vi "save_max_p_Data.vi"(0 "Experiment Indicator":string, 1 "Cell details cluster":T3={"Cell Position"=16, "Cell Label"="", "Pixel to measure"=0, "Area (cm^2)"=0.126, "Variable"="", "Variable value"="", "Scan settings in queue"=0, "Light or dark"="", "Measurement Type"=""} {"Pixel to measure" items=["All", "1", "2", "3", "4", "5", "6", "7", "8"]}, 3 "Intensity (no. of suns)":string, 4 "Data Array":dbl[][](array[numeric]), 6 "Username":string, 7 "Scan settings":T1={"J-V scan"=TRUE, "J-t scan"=FALSE, "Min voltage (V)"=0.0, "Max voltage (V)"=1.4, "Step (V)"=0.01, "Measurement delay (ms)"=10.0, "1st scan FB-SC"=TRUE, "Inverted structure"=FALSE, "Stabilisation time (s)"=0.0, "Stabilisation mode"=0, "Stabilisation value (V or A) "=0.0, "Step time (s)"=1.0, "Integration time"=0, "Repeat light scans"=FALSE, "Stabilisation in the dark?"=FALSE, "J-t Min (V)"=0.0, "J-t Max (V)"=1.4, "J-t Step (V)"=0.01, "Max. power stabilisation"=FALSE, "J-t 1st scan FB-SC"=TRUE, "J-t Inverted structure"=FALSE, "Max power tracking"=FALSE, "Vmp (V)"=0.7, "Total stabilisation time (s)"=100.0, "J-t best pixel only"=0, "Max power best pixel only"=0, "Vmp from J-V scan"=FALSE, "No. of repeat scans"=2.0, "Only repeat for best pixel"=0, "Stabilisation time step (s)"=1.0, "Illumination conditions"=2, "Scan rate min (V/s)"=0.1, "Scan rate max (V/s)"=1.0, "No. of scan rate steps"=1.0, "Scan rate voltage step priority"=FALSE, "Scan rate measurement delay priority"=FALSE, "J-t Illumination conditions"=0, "Max P stab. Specific voltage"=FALSE} {"J-t Illumination conditions" items=["Light only", "Dark only", "Light then dark", "Dark then light"]; "No. of scan rate steps" min=1.0 step=1.0; "Illumination conditions" items=["Light only", "Dark only", "Light then dark", "Dark then light", "Light then dark then light", "Dark then light then dark"]; "Only repeat for best pixel" items=["only for best pixel", "for best 2 pixels", "for best 3 pixels", "for best 4 pixels", "for best 5 pixels", "for best 6 pixels", "for best 7 pixels", "for all pixels"]; "No. of repeat scans" min=1.0 step=1.0; "Max power best pixel only" items=["only the best pixel", "the best 2 pixels", "the best 3 pixels", "the best 4 pixels", "the best 5 pixels", "the best 6 pixels", "the best 7 pixels", "all pixels"]; "J-t best pixel only" items=["only the best pixel", "the best 2 pixels", "the best 3 pixels", "the best 4 pixels", "the best 5 pixels", "the best 6 pixels", "the best 7 pixels", "all pixels"]; "Integration time" items=["Fast", "Normal", "High Accuracy"]; "Stabilisation mode" items=["V", "I"]; "Measurement delay (ms)" min=10.0}, 10 "Date array":string[](array[string])) -> (14 "Master Log":string[][](table), 15 "File path for master log":path, 17 "File path for Jt data":path, 18 "File path for Jt image":path)   [LabVIEW 2016]
uses:
  TypeDefs/scan_settings.ctl
  TypeDefs/Settings Boolean.ctl
  <vilib>/Utility/file.llb/Write Delimited Spreadsheet (string).vi
  <vilib>/Utility/file.llb/Read Delimited Spreadsheet (string).vi
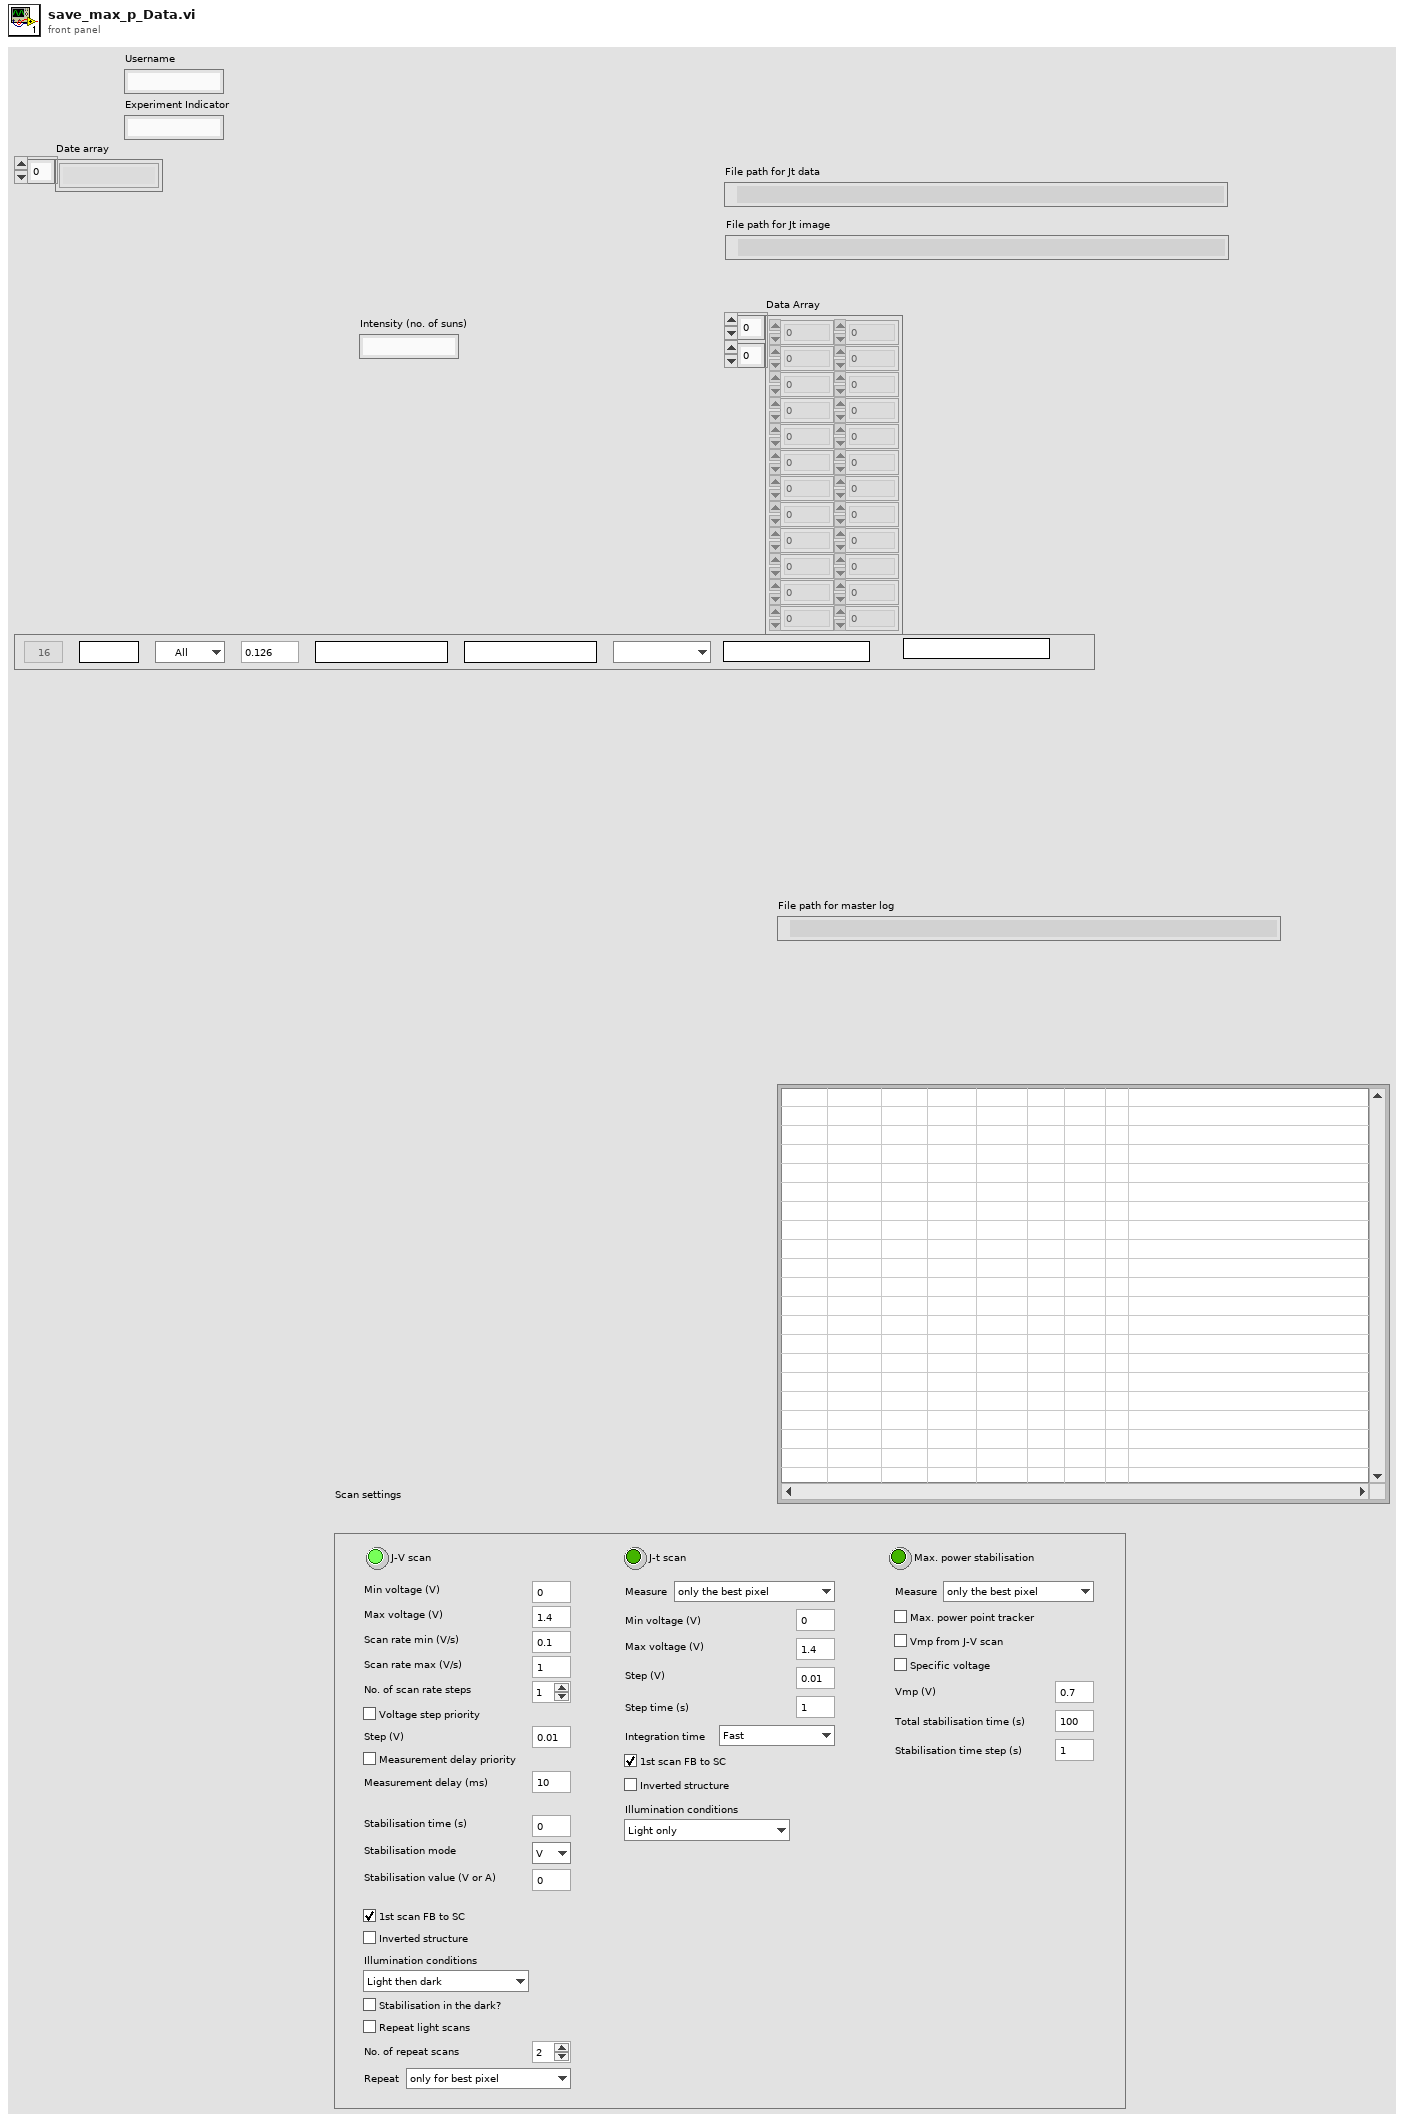
[diagram p1: front panel]
types:
  T1 = typedef "scan_settings.ctl" = cluster{"J-V scan":T2, "J-t scan":bool, "Min voltage (V)":dbl, "Max voltage (V)":dbl, "Step (V)":dbl, "Measurement delay (ms)":dbl, "1st scan FB-SC":bool, "Inverted structure":bool, "Stabilisation time (s)":dbl, "Stabilisation mode":u16, "Stabilisation value (V or A) ":dbl, "Step time (s)":dbl, "Integration time":u16, "Repeat light scans":bool, "Stabilisation in the dark?":bool, "J-t Min (V)":dbl, "J-t Max (V)":dbl, "J-t Step (V)":dbl, "Max. power stabilisation":bool, "J-t 1st scan FB-SC":bool, "J-t Inverted structure":bool, "Max power tracking":bool, "Vmp (V)":dbl, "Total stabilisation time (s)":dbl, "J-t best pixel only":u16, "Max power best pixel only":u16, "Vmp from J-V scan":bool, "No. of repeat scans":dbl, "Only repeat for best pixel":u16, "Stabilisation time step (s)":dbl, "Illumination conditions":u16, "Scan rate min (V/s)":dbl, "Scan rate max (V/s)":dbl, "No. of scan rate steps":dbl, "Scan rate voltage step priority":bool, "Scan rate measurement delay priority":bool, "J-t Illumination conditions":u16, "Max P stab. Specific voltage":bool}
  T2 = typedef "Settings Boolean.ctl" = bool
  T3 = cluster{"Cell Position":i32, "Cell Label":string, "Pixel to measure":u16, "Area (cm^2)":dbl, "Variable":string, "Variable value":string, "Scan settings in queue":u16, "Light or dark":string, "Measurement Type":string}
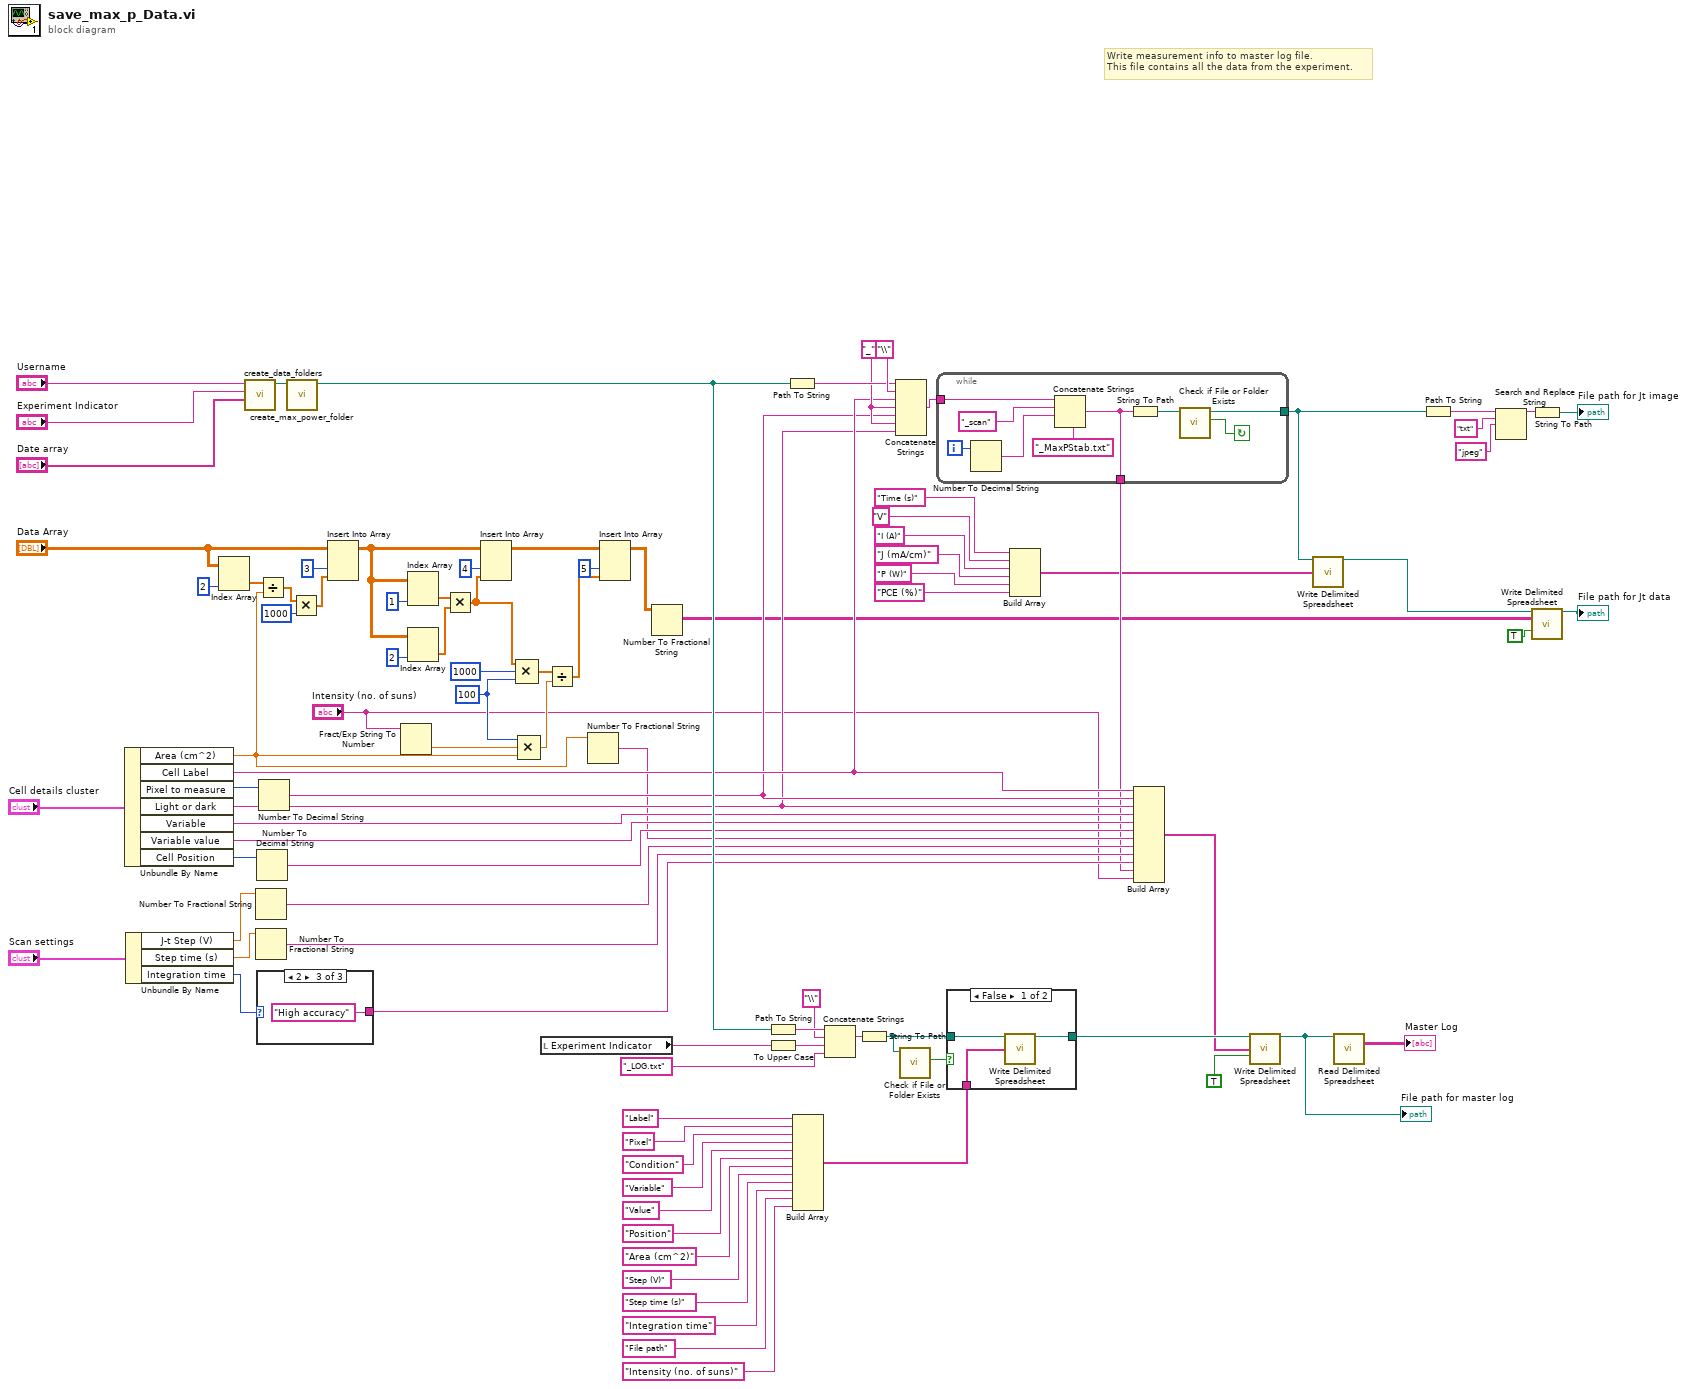
[diagram p0: block diagram]
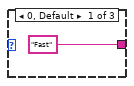
[diagram p2: hidden frame]
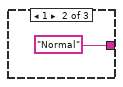
[diagram p3: hidden frame]
diagram:
  w58 = 100
  w84 = "_"
  # "Write measurement info to master log file.\nThis file contains all the data from the experiment."
  n1 = Unbundle By Name("Cell details cluster") -> ("Area (cm^2)"=w12:dbl, "Cell Label"=w19:string, "Pixel to measure"=w80:u16, "Light or dark"=w17:string, "Variable"=w16:string, "Variable value"=w15:string, "Cell Position"=w14:i32)
  n2 = Unbundle By Name("Scan settings") -> ("J-t Step (V)"=w22:dbl, "Step time (s)"=w10:dbl, "Integration time"=w23:u16)
  n3 = Index Array(array="Data Array", index (col)=2) -> (element=w83:dbl[])  [unwired: 1 in]
  n4 = call "create_data_folders.vi"("Date array"="Date array", "Experiment Indicator"="Experiment Indicator", "username"="Username") -> ("Data Output Folder"=w49:path)  [unwired: 8 in]
  n5 = Number To Fractional String(number=w22) -> (F-format string=w9:string)  [unwired: 3 in]
  n6 = Number To Fractional String(number=w10) -> (F-format string=w8:string)  [unwired: 3 in]
  n7 = Number To Decimal String(number=w14) -> (decimal integer string=w13:string)  [unwired: 1 in]
  n8 = case shown="2" w23 {
    tunnel: ["Fast" "Normal" "High accuracy"] -> w7
    frame 0, Default {
    }
    frame 1 {
    }
    frame 2 {
    }
  }
  n9 = Divide(x=w83, y=w12) -> (x/y=w78:dbl[])
  n10 = Number To Decimal String(number=w80) -> (decimal integer string=w18:string)  [unwired: 1 in]
  n11 = call "create_max_power_folder.vi"("Data Folder In"=w49) -> ("Data Output Folder"=w21:path)  [unwired: 10 in]
  n12 = Multiply(x=w78, y=1000) -> (x*y=w79:dbl[])
  n13 = Insert Into Array(array="Data Array", index (col)=3, new element=w79) -> (w63:dbl[][])  [unwired: 1 in]
  n14 = Fract/Exp String To Number(string="Intensity (no. of suns)") -> (number=w57:dbl)  [unwired: 3 in, 1 out]
  n15 = Index Array(array=w63, index (col)=1 ("disabled index (col)")) -> (element=w68:dbl[])  [unwired: 1 in]
  n16 = Index Array(array=w63, index (col)=2 ("disabled index (col)")) -> (element=w67:dbl[])  [unwired: 1 in]
  n17 = Multiply(x=w68, y=w67) -> (x*y=w50:dbl[])
  n18 = Insert Into Array(array=w63, index (col)=4 ("disabled index (col)"), new element=w50) -> (w62:dbl[][])  [unwired: 1 in]
  n19 = Compound Arithmetic op=MULTIPLY(w50, 1000, w58) -> (w59:dbl[])
  n20 = Compound Arithmetic op=MULTIPLY(w58, w57, w12) -> (w56:dbl)
  n21 = local read "Experiment Indicator"() -> (w20:string)
  n22 = Divide(x=w59, y=w56) -> (x/y=w55:dbl[])
  n23 = Number To Fractional String(number=w12) -> (F-format string=w11:string)  [unwired: 3 in]
  n24 = Insert Into Array(array=w62, index (col)=5 ("disabled index (col)"), new element=w55) -> (w54:dbl[][])  [unwired: 1 in]
  n25 = Number To Fractional String(number=w54) -> (F-format string=w1:string[][])  [unwired: 3 in]
  n26 = Path To String(path=w21) -> (string=w47:string)
  n27 = To Upper Case(1:w20) -> (0:w41:string)
  n28 = Path To String(path=w21) -> (string=w94:string)
  n29 = Build Array("Label", "Pixel", "Condition", "Variable", "Value", "Position", "Area (cm^2)", "Step (V)", "Step time (s)", "Integration time", "File path", "Intensity (no. of suns)") -> (w25:string[])
  n30 = Concatenate Strings(w47, "\\", w41, "_LOG.txt") -> (w45:string)
  n31 = String To Path(string=w45) -> (path=w39:path)
  n32 = Concatenate Strings(w94, "\\", w19, w84, w18, w84, w17) -> (w86:string)
  n33 = call <vilib>:"Check if File or Folder Exists.vi"("path"=w39) -> ("file or folder exists?"=w40:bool)  [unwired: 8 in, 2 out]
  n34 = while {
    tunnel: w86 -> [w107]
    tunnel: [w100] -> w76
    tunnel: [w99] -> w6
    i -> [w105]
    stop <- w101 continue-if-true
    n35 = Number To Decimal String(number=w105) -> (decimal integer string=w104:string)  [unwired: 1 in]
    n36 = Concatenate Strings(w107, "_scan", w104, "_MaxPStab.txt") -> (w99:string)
    n37 = String To Path(string=w99) -> (path=w102:path)
    n38 = call <vilib>:"Check if File or Folder Exists.vi"("path"=w102) -> ("file or folder exists?"=w101:bool, "dup path"=w100:path)  [unwired: 8 in, 1 out]
  }
  n39 = case shown="False" w40 {
    tunnel: w39 -> [w110 w111]
    tunnel: [w109 w111] -> w38
    tunnel: w25 -> [w108 _]
    frame False {
      n40 = call-poly <vilib>:"Write Delimited Spreadsheet.vi"("file path (dialog if empty)"=w110, "1D data"=w108) -> ("new file path (Not A Path if cancelled)"=w109:path)  [unwired: 12 in, 1 out]
    }
    frame True {
    }
  }
  n41 = Build Array("Time (s)", "V", "I (A)", "J (mA/cm)", "P (W)", "PCE (%)") -> (w2:string[])
  n42 = Build Array(w19, w18, w17, w16, w15, w13, w11, w9, w8, w7, w6, "Intensity (no. of suns)") -> (w4:string[])
  n43 = call-poly <vilib>:"Write Delimited Spreadsheet.vi"("file path (dialog if empty)"=w38, "1D data"=w4, "append to file? (new file:F)"=TRUE) -> ("new file path (Not A Path if cancelled)"=w43:path)  [unwired: 11 in, 1 out]
  "File path for master log" <- w43
  n44 = call-poly <vilib>:"Write Delimited Spreadsheet.vi"("file path (dialog if empty)"=w76, "1D data"=w2) -> ("new file path (Not A Path if cancelled)"=w75:path)  [unwired: 12 in, 1 out]
  n45 = call-poly <vilib>:"Read Delimited Spreadsheet.vi"("file path (dialog if empty)"=w43) -> ("all rows"=→"Master Log":string[][])  [unwired: 9 in, 5 out]
  n46 = Path To String(path=w76) -> (string=w85:string)
  n47 = Search and Replace String(input string=w85, search string="txt", replace string="jpeg") -> (result string=w93:string)  [unwired: 5 in, 3 out]
  n48 = String To Path(string=w93) -> (path=→"File path for Jt image":path)
  n49 = call-poly <vilib>:"Write Delimited Spreadsheet.vi"("file path (dialog if empty)"=w75, "2D data"=w1, "append to file? (new file:F)"=TRUE) -> ("new file path (Not A Path if cancelled)"=→"File path for Jt data":path)  [unwired: 11 in, 1 out]
